vi "DriveUntilY.vi"(7 "Stop  Distance":dbl, 8 "error in":errorcluster, 9 "y":dbl, 10 "x":dbl) -> (0 "error out":errorcluster)   [LabVIEW 2017]
uses:
  Robot Global Data.vi
panel:
  # "DriveUntilY Autonomous Commands\nTeam 34 Rockets"
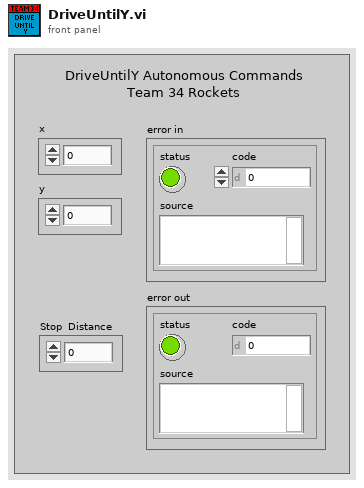
[diagram p1: front panel]
types:
  T1 = typedef "WPI_EncoderDevRef.ctl" = cluster{"DevStatus":errorcluster, "EncoderIndex":T2, "CounterIndex":T3, "DistancePerCount":dbl, "Decoding Type":T4}
  T2 = typedef "FPGA_EncoderIdx.ctl" = enum8{"Enc 0", "Enc 1", "Enc 2", "Enc 3", "Enc 4", "Enc 5", "Enc 6", "Enc 7", "Invalid"}
  T3 = typedef "FPGA_CounterCtrSystemIndex.ctl" = enum8{"Ctr 0", "Ctr 1", "Ctr 2", "Ctr 3", "Ctr 4", "Ctr 5", "Ctr 6", "Ctr 7", "Invalid"}
  T4 = typedef "WPI_EncoderType.ctl" = enum16{"1x", "2x", "4x"}
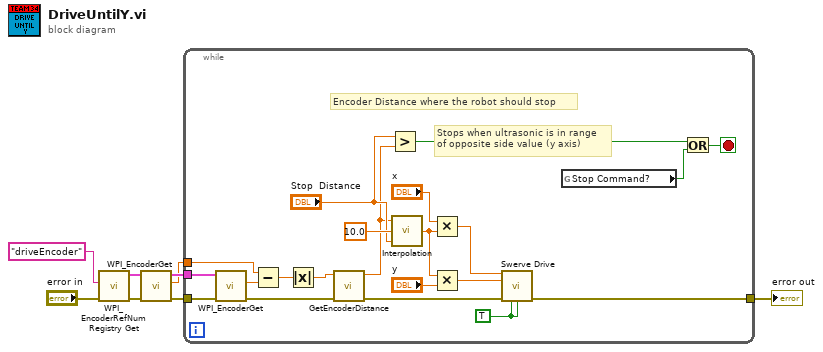
[diagram p0: block diagram]
diagram:
  n1 = call <vilib>:"WPI_EncoderRefNum Registry Get.vi"("error in (no error)"="error in", "refnum name"="driveEncoder") -> ("error out"=w4:errorcluster, "EncoderDevRef"=w5:T1)  [unwired: 8 in]
  n2 = call <vilib>:"WPI_EncoderGet.vi"("error in (no error)"=w4, "EncoderDevRef"=w5) -> ("error out"=w3:errorcluster, "Distance"=w1:dbl, "EncoderDevRef"=w2:T1)  [unwired: 4 in, 3 out]
  n3 = while {
    tunnel: w3 -> [w17]
    tunnel: w2 -> [w20]
    tunnel: [w27] -> w8
    tunnel: w1 -> [w16]
    stop <- w28 stop-if-true
    w26 = TRUE ("Autonomous?")
    # "Encoder Distance where the robot should stop"
    # "Stops when ultrasonic is in range\nof opposite side value (y axis)"
    n4 = call <vilib>:"WPI_EncoderGet.vi"("error in (no error)"=w17, "EncoderDevRef"=w20) -> ("error out"=w19:errorcluster, "Distance"=w15:dbl)  [unwired: 4 in, 4 out]
    n5 = Subtract(x=w16, y=w15) -> (x-y=w14:dbl)
    n6 = Absolute Value(x=w14) -> (abs(x)=w13:dbl)
    n7 = call "GetEncoderDistance.vi"("Error In"=w19, "Distance"=w13) -> ("Error Out"=w18:errorcluster, "Distance Travelled (in)"=w9:dbl)  [unwired: 8 in]
    n8 = Greater?(x="Stop  Distance", y=w9) -> (0:w11:bool)
    n9 = call "Interpolation.vi"("Distance Objective"="Stop  Distance", "Start Distance"=10.0, "Current Encoder Distance"=w9) -> ("Motor Output"=w21:dbl)
    n10 = Multiply(x="x", y=w21) -> (x*y=w24:dbl)
    n11 = Multiply(x=w21, y="y") -> (x*y=w22:dbl)
    n12 = call "Swerve Drive.vi"("X"=w24, "Y"=w22, "Error In"=w18, "Robot Centric?"=w26, "Autonomous?"=w26) -> ("Error Out"=w27:errorcluster)  [unwired: 6 in, 4 out]
    n13 = global read "Robot Global Data.vi" "Stop Command?"() -> (w29:bool)
    n14 = Or(x=w11, y=w29) -> (x .or. y?=w28:bool)
  }
  "error out" <- w8
